vi "I2C Read.vi"(8 "error in (no error)":errorcluster, 9 "pdata":string, 10 "intAddress":u8, 11 "deviceID":u8) -> (0 "error out":errorcluster, 1 "pdata out":string, 3 "function return":u32)   [LabVIEW 2014, in "atmcd32d.lvlib"]
doc: "unsigned int WINAPI I2CRead(BYTE deviceID, BYTE intAddress, BYTE * pdata);"
uses:
  atmcd32d.lvlib
  atmcd32d.dll
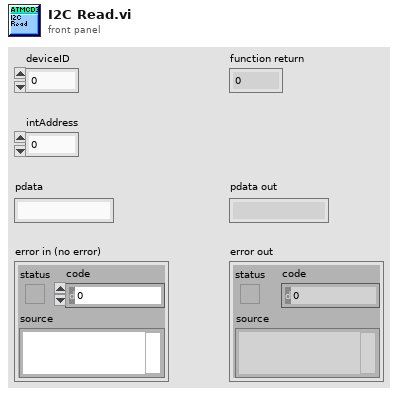
[diagram p1: front panel]
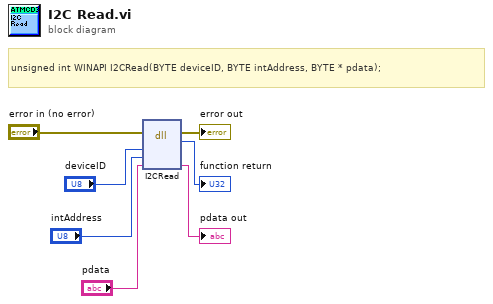
[diagram p0: block diagram]
diagram:
  # "unsigned int WINAPI I2CRead(BYTE deviceID, BYTE intAddress, BYTE * pdata);"
  n1 = dll-call lib="C:/Users/Bakir/Documents/Lambda2-Testing/lib/Andorlib/atmcd32d.*" fn="I2CRead"(error in="error in (no error)", "deviceID"="deviceID", "intAddress"="intAddress", "pdata"="pdata") -> (error out=→"error out":errorcluster, →"function return":u32, "pdata"=→"pdata out":string)  [unwired: 4 in, 1 out]
